vi "NI VeriStand - Get Alias List.vi"(8 "error in (no error)":errorcluster, 11 "WorkspaceManager in":T1) -> (0 "error out":errorcluster, 1 "Channels":string[](array[string]), 2 "Aliases":string[](array[string]), 3 "WorkspaceManager out":T1)   [LabVIEW 2020, in "NI_VS Workspace ExecutionAPI.lvlib"]
doc: "Returns lists of all the defined aliases and their corresponding channels."
uses:
  <vilib>/NI VeriStand/Execution/Workspace/NI_VS Workspace ExecutionAPI.lvlib
  <vilib>/NI VeriStand/Execution/Workspace/WorkspaceAPI.ctl
  NationalInstruments.VeriStand.ClientAPI
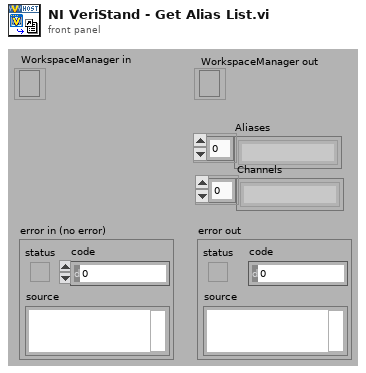
[diagram p1: front panel]
types:
  T1 = typedef "NI_VS Workspace ExecutionAPI.lvlib/WorkspaceAPI.ctl" = refnum<k24>
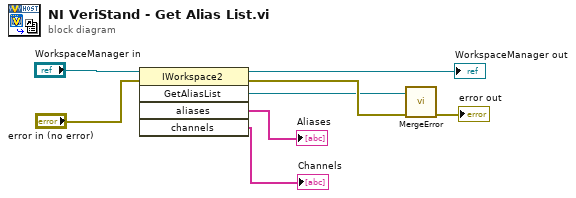
[diagram p0: block diagram]
diagram:
  n1 = invoke class="IWorkspace2" method="GetAliasList"(reference="WorkspaceManager in", error in="error in (no error)") -> (reference out=→"WorkspaceManager out":T1, error out=w6:errorcluster, "GetAliasList"=w5:refnum<k24>, "aliases"=→"Aliases":string[], "channels"=→"Channels":string[])  [unwired: 3 in]
  n2 = call <vilib>:"MergeError.vi"("error in (no error)"=w6, "Error"=w5) -> ("error out"=→"error out":errorcluster)  [unwired: 9 out]
